vi "PH_Beamline_Chief.destructor.vi"(0 "i ref in":refnum<vi>, 5 "error in(no error)":errorcluster) -> (19 "error out":errorcluster)   [LabVIEW 2014, in "PH_Beamline_Chief.lvlib"]
doc: "This is the destructor of a class.\n\nLicense Agreement for this software:\n\nCopyright (C)\nGesellschaft für Schwerionenforschung, GSI\nPlanckstr. 1\n64291 Darmstadt\nGermany\n\nContact: D.Beck@gsi.de \n\nThis program is free software; you can redistribute it and/or modify it under the terms of the \nGNU General Public License as published by the Free Software Foundation; either version 2 of \nthe license, or (at your option) any later version.\n\nThis program is distributed in the hope that it will be useful, but WITHOUT ANY WARRANTY; \nwithout even the implied warranty of MERCHANTABILITY or FITNESS FOR A PARTICULAR PURPOSE. See the GNU General License for more details (http://www.gnu.org).\n\nGesellschaft für Schwerionenforschung, GSI\nPlanckstr. 1, 64291 Darmstadt, Germany\nFor all questions and ideas contact: M.Richter@gsi.de, H.Brand@gsi.de or D.Beck@gsi.de.\nLast update: 16-JUN-2004"
uses:
  PH_Beamline_Chief.lvlib
  CSlibraries-extern/DimLVEvent/LVDimInterface/LVDimInterface.lvlib
  PH_Beamline/PH_Beamline.lvlib
  PH_BL-Master/PH_BL-Master.lvlib
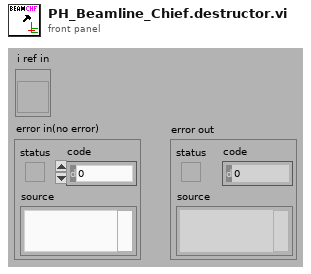
[diagram p1: front panel]
types:
  T1 = typedef "PH_Beamline_Chief.lvlib/PH_Beamline_Chief.i attribute.ctl" = cluster{"BL Service IDs":cluster{"YLF_BL_Status":i32, "fs_BL_Status":i32, "fs_YLF_BL_Status":i32, "ns_BL_Status":i32, "PA_Input_BL_Status":i32, "PA_UnDelay_BL_Status":i32, "PA_Delay_BL_Status":i32, "PA_BL_Status":i32, "PA_Bypass_BL_Status":i32, "PA_Exit_BL_Status":i32, "PA_LL_BL_Status":i32, "LL_BL_Status":i32, "PA_MA_BL_Status":i32, "MA_Exit_BL_Status":i32, "MA_Z6_BL_Status":i32, "Z6_BL_Status":i32, "MA_LB_BL_Status":i32, "LB_TB2_BL_Status":i32, "PA_before_Bypass_BL_Status":i32, "LB_TB3_BL_Status":i32}, "R2S Service ID":i32, "Settings":cluster{"Wanted":T2, "GUI Ref":refnum<vi>, "Service ID":i32}}
  T2 = typedef "PH_Beamline_Chief.lvlib/PH_Beamline_Chief.Settings.ctl" = cluster{"PA Doublepass Mode":bool, "Compressor Vaccuum LB not relevant":bool, "Windowshutter TB2 not relevant":bool, "Windowshutter TB3 not relevant":bool}
  T3 = enum16{"SetAttribute", "GetAttribute", "CreateAttribute", "DestroyAttribute", "DestroyAllAtributes"}
  T4 = cluster{"YLF_BL_Status":i32, "fs_BL_Status":i32, "fs_YLF_BL_Status":i32, "ns_BL_Status":i32, "PA_Input_BL_Status":i32, "PA_UnDelay_BL_Status":i32, "PA_Delay_BL_Status":i32, "PA_BL_Status":i32, "PA_Bypass_BL_Status":i32, "PA_Exit_BL_Status":i32, "PA_LL_BL_Status":i32, "LL_BL_Status":i32, "PA_MA_BL_Status":i32, "MA_Exit_BL_Status":i32, "MA_Z6_BL_Status":i32, "Z6_BL_Status":i32, "MA_LB_BL_Status":i32, "LB_TB2_BL_Status":i32, "PA_before_Bypass_BL_Status":i32, "LB_TB3_BL_Status":i32}
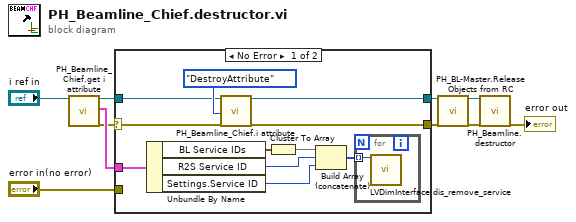
[diagram p0: block diagram]
diagram:
  n1 = call "PH_Beamline_Chief.get i attribute.vi"("i ref in"="i ref in") -> ("i ref out"=w8:refnum<vi>, "i attribute"=w10:T1, "error out"=w7:errorcluster)  [unwired: 16 in]
  n2 = case shown="No Error" w7 {
    selector: w7 -> [w12 _]
    tunnel: w10 -> [w20 _]
    tunnel: w8 -> [w13 w24]
    tunnel: [w17 w24] -> w3
    tunnel: [w16 w23] -> w1
    tunnel: "error in(no error)" -> [_ w23]
    frame No Error {
      n3 = Unbundle By Name(w20) -> ("BL Service IDs"=w19:T4, "R2S Service ID"=w14:i32, "Settings.Service ID"=w11:i32)
      n4 = call "PH_Beamline_Chief.i attribute.vi"("VI Refnum"=w13, "Action"=T3."DestroyAttribute", "error in (no error)"=w12) -> ("VI Refnum out"=w17:refnum<vi>, "error out"=w16:errorcluster)  [unwired: 14 in, 1 out]
      n5 = Cluster To Array(cluster=w19) -> (array=w18:i32[])
      n6 = Build Array (concatenate)(w18, w14, w11) -> (w15:i32[])
      n7 = for {
        tunnel: w15 -> [w22] mode=indexing
        n8 = call "LVDimInterface.dis_remove_service.vi"("my_serviceID"=w22) -> ()  [unwired: 18 in, 1 out]
      }
    }
    frame Error {
    }
  }
  n9 = call "PH_BL-Master.Release Objects from RC.vi"("VI in"=w3, "error in (no error)"=w1) -> ("VI out"=w4:refnum<vi>, "error out"=w2:errorcluster)  [unwired: 16 in]
  n10 = call "PH_Beamline.destructor.vi"("i ref in"=w4, "error in(no error)"=w2) -> ("error out"=→"error out":errorcluster)  [unwired: 17 in]
